vi "ConfigWFG.vi"(0 "object in":refnum<class "AD2andExtAWG.lvclass">, 2 "Config(var)":variant, 5 "error in (no error)":errorcluster) -> (14 "object out":refnum<class "AD2andExtAWG.lvclass">, 19 "error out":errorcluster)   [LabVIEW 2019, in "AD2andExtAWG.lvclass"]
uses:
  AD2andExtAWG.lvclass
  AD2andExtAWG.lvclass/AD2andExtAWG.ctl
  AFG3022B_class/AFG3022B.lvclass
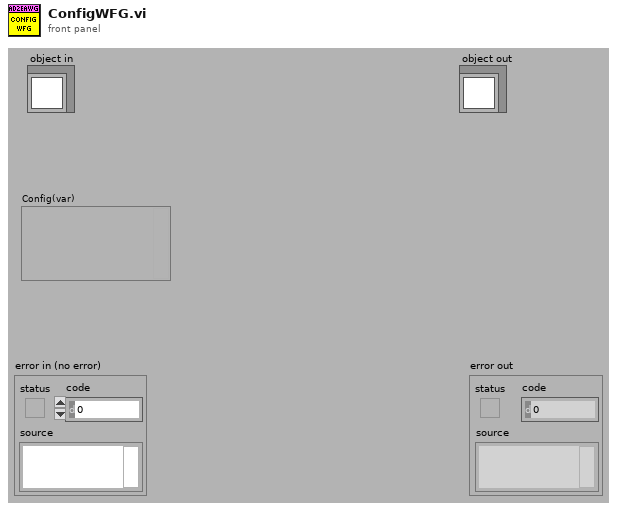
[diagram p1: front panel]
types:
  T1 = cluster{"ConfigDataCh1":cluster{"Frequency Hz (1000 Hz)":dbl, "Waveform Function (0: Sine)":u16, "Amplitude (1 Vpp)":dbl, "DC Offset (0.00 V)":dbl, "Phase Level (-1)":dbl, "Phase Unit (0: Radian)":u16}, "ConfigDataCh2":cluster{"Frequency Hz (1000 Hz)":dbl, "Waveform Function (0: Sine)":u16, "Amplitude (1 Vpp)":dbl, "DC Offset (0.00 V)":dbl, "Phase Level (-1)":dbl, "Phase Unit (0: Radian)":u16}}
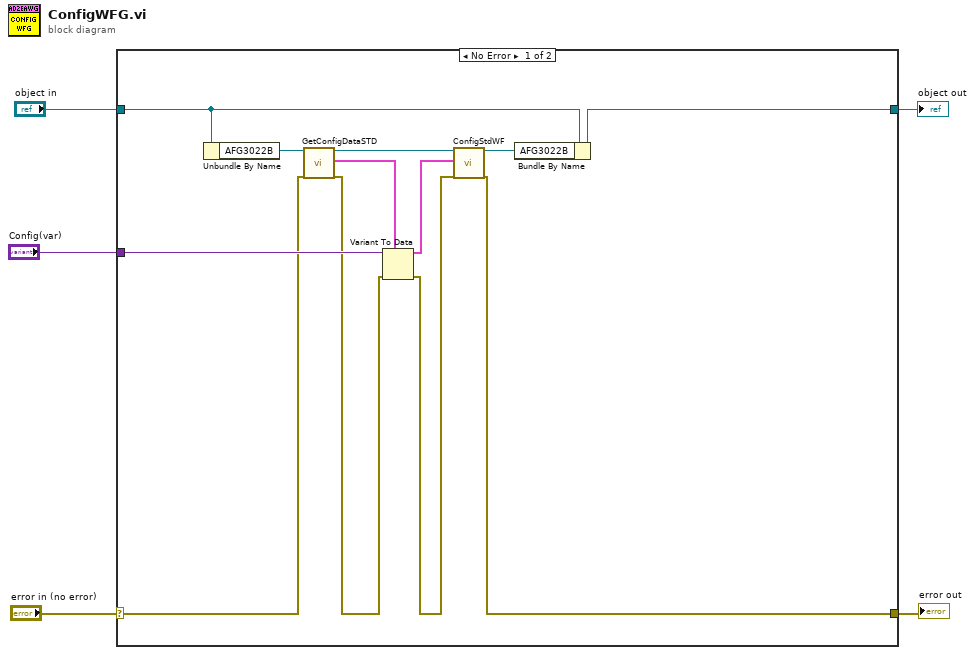
[diagram p0: block diagram]
diagram:
  n1 = case shown="No Error" "error in (no error)" {
    selector: "error in (no error)" -> [w13 w19]
    tunnel: [w9 w19] -> w4
    tunnel: [w8 w18] -> w2
    tunnel: "object in" -> [w17 w18]
    tunnel: "Config(var)" -> [w14 _]
    frame No Error {
      n2 = Unbundle By Name(w17) -> ("AFG3022B"=w16:refnum<class "AFG3022B.lvclass">)
      n3 = call-dynamic "GetConfigDataSTD.vi"("object in"=w16, "error in (no error)"=w13) -> ("object out"=w15:refnum<class "AFG3022B.lvclass">, "Configdatastd"=w6:T1, "error out"=w11:errorcluster)  [unwired: 15 in]
      n4 = Variant To Data(error in=w11, type=w6, Variant=w14) -> (data=w12:T1, error out=w10:errorcluster)
      n5 = call-dynamic "ConfigStdWF.vi"("object in"=w15, "Configdatastd"=w12, "error in (no error)"=w10) -> ("object out"=w7:refnum<class "AFG3022B.lvclass">, "error out"=w9:errorcluster)  [unwired: 15 in]
      n6 = Bundle By Name(cluster=w17, "AFG3022B"=w7) -> (w8:refnum<class "AD2andExtAWG.lvclass">)
    }
    frame Error {
    }
  }
  "error out" <- w4
  "object out" <- w2
